vi "Untitled 3.vi"() -> ()   [LabVIEW 2016]
uses:
  <vilib>/Analysis/baseanly.llb/Mean (DBL).vi
  <vilib>/Analysis/NI_AALBase.lvlib
panel:
  out "output variable":dbl
  in  "stop":bool
  out "output variable 2":dbl
  out "Waveform Chart 2":dbl(graph)
  out "Numeric 2":dbl
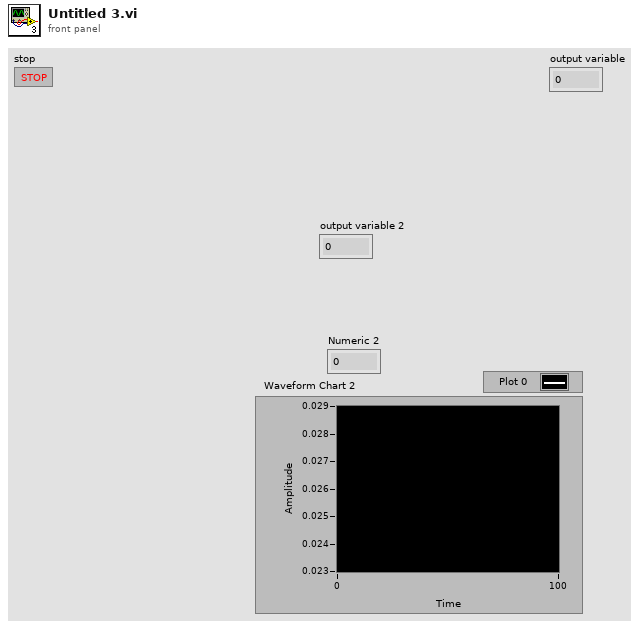
[diagram p1: front panel]
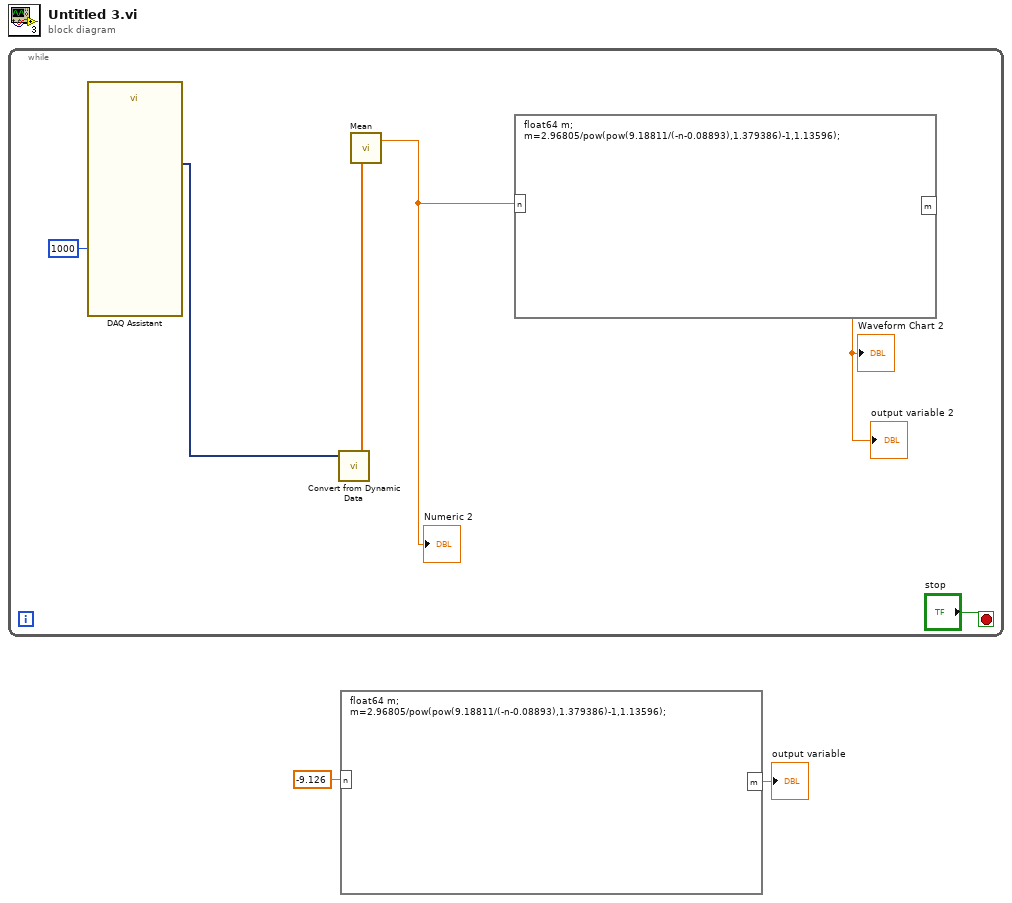
[diagram p0: block diagram]
diagram:
  n1 = while {
    stop <- "stop" stop-if-true
    n2 = call "DAQ Assistant"("number of samples"=1000) -> ("data"=w5:dynamicdata)  [unwired: 16 in, 2 out]
    n3 = call "Convert from Dynamic Data"("Dynamic Data Type"=w5) -> ("Array"=w8:dbl[])  [unwired: 3 in]
    n4 = call-poly <vilib>:"Mean.vi"("X"=w8) -> ("mean"=w6:dbl)  [unwired: 1 out]
    "Numeric 2" <- w6
    n5 = formula code="float64 m;\nm=2.96805/pow(pow(9.18811/(-n-0.08893),1.379386)-1,1.13596);"("n"=w6) -> ("m"=→"Waveform Chart 2" →"output variable 2":dbl)
  }
  n6 = formula code="float64 m;\nm=2.96805/pow(pow(9.18811/(-n-0.08893),1.379386)-1,1.13596);"("n"=-9.126 ("input variable")) -> ("m"=→"output variable":dbl)
